vi "test SSL Client No Listener.vi"(8 "error in (no error)":errorcluster, 11 "TestCase in":refnum<class "test SSL Client.lvclass">) -> (0 "error out":errorcluster, 3 "TestCase out":refnum<class "test SSL Client.lvclass">)   [LabVIEW 2013, in "test SSL Client.lvclass"]
uses:
  test SSL Client.lvclass
  <vilib>/addons/_JKI Toolkits/VI Tester/TestCase.llb/TestCase.lvclass
  SSL_Lib/BIO/BIO.lvclass
  SSL_Lib/SSL-Context/SSL-Context.lvclass
  SSL_Lib/SSL/SSL.lvclass
  SSL_Lib/SSL/SSL_Mode.ctl
  suite SSL Client/suite SSL Client/SSL Context.vi
  suite SSL Client/suite SSL Client/suite SSL Client.lvclass
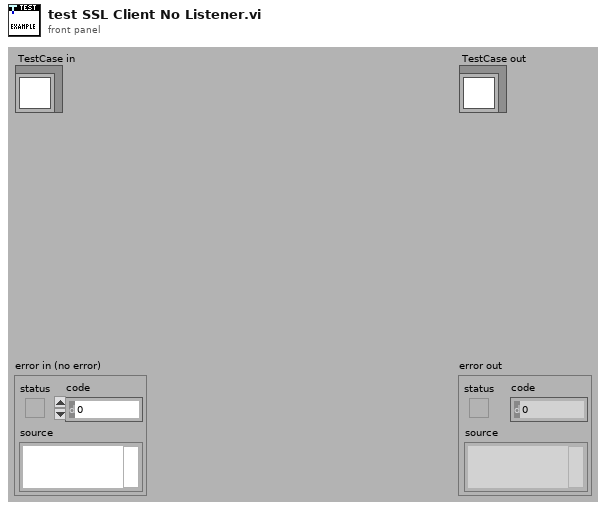
[diagram p1: front panel]
types:
  T1 = typedef "SSL_Lib.lvlib/SSL.lvclass/SSL_Mode.ctl" = i32
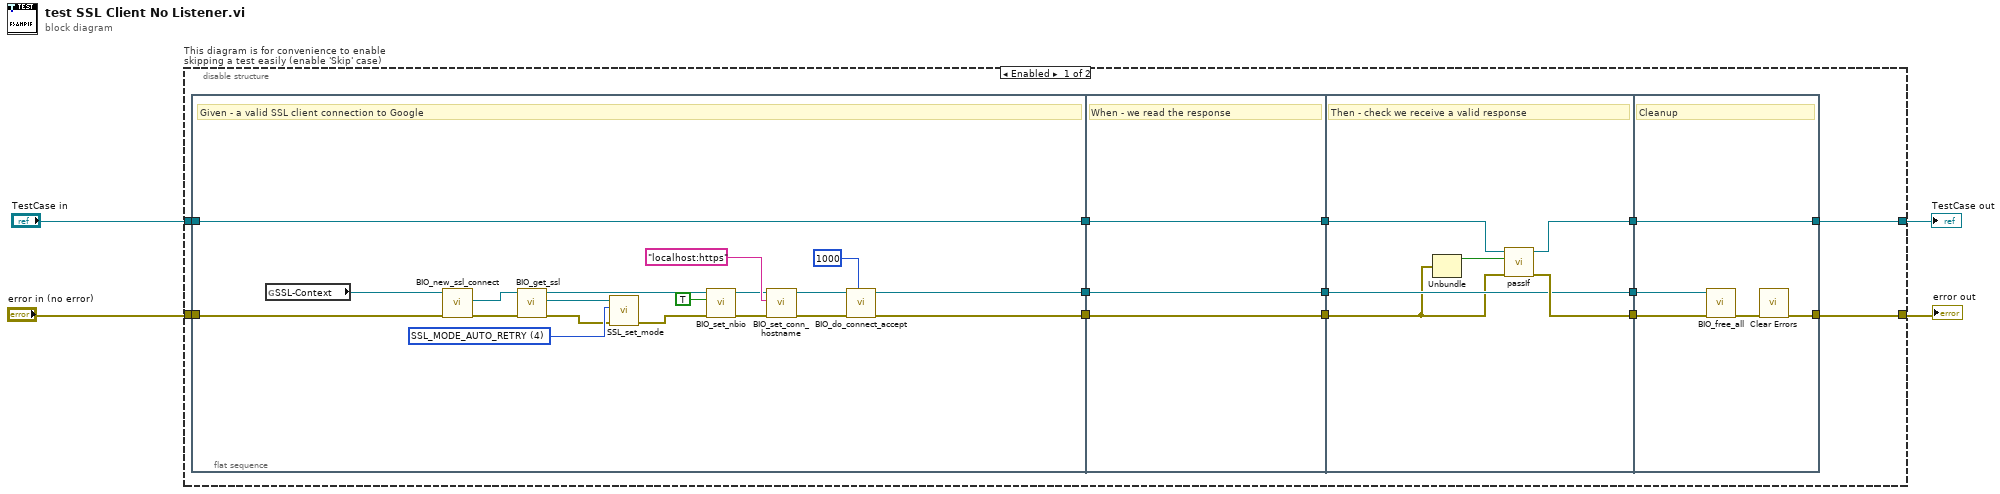
[diagram p0: block diagram]
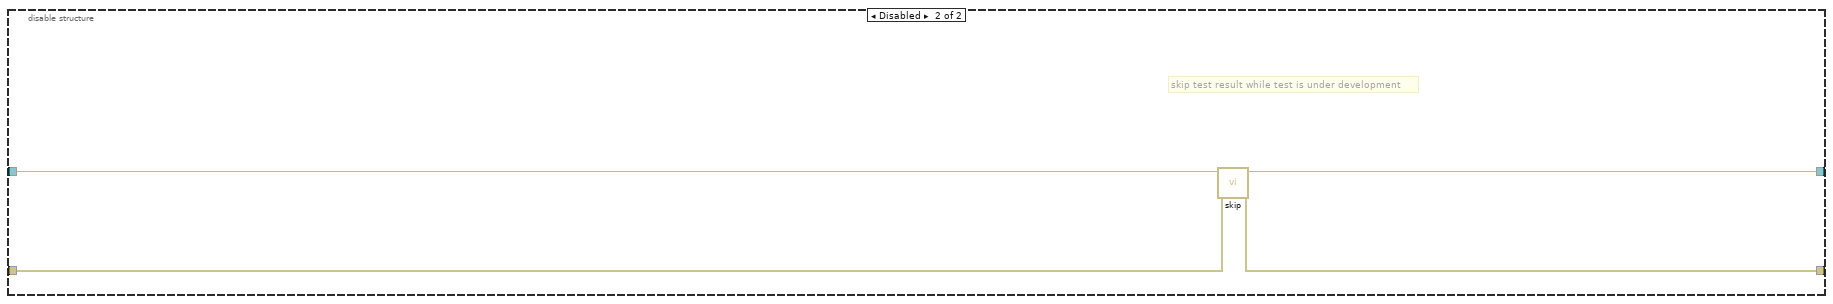
[diagram p2: hidden frame]
diagram:
  n1 = disable-structure "This diagram is for convenience to enable skipping a test easily (enable 'Skip' case)" shown="Enabled" {
    disable-tunnel: "TestCase in" -> [w12 w54]
    disable-tunnel: [w11 w52] -> w1
    disable-tunnel: [w10 w53] -> w3
    disable-tunnel: "error in (no error)" -> [w13 w51]
    frame Enabled {
      n2 = flat-sequence {
        tunnel: w13 -> [w26]
        tunnel: w12 -> [w33]
        tunnel: [w33] -> w17
        tunnel: [w19] -> w7
        tunnel: [w18] -> w6
        tunnel: [w39] -> w16
        tunnel: w17 -> [w39]
        tunnel: [w37] -> w9
        tunnel: w7 -> [w38]
        tunnel: w6 -> [w37]
        tunnel: [w38] -> w5
        tunnel: [w44] -> w15
        tunnel: [w43] -> w14
        tunnel: w16 -> [w45]
        tunnel: w9 -> [w42]
        tunnel: [w42] -> w8
        tunnel: w5 -> [w41]
        tunnel: [w46] -> w10
        tunnel: [w50] -> w11
        tunnel: w15 -> [w50]
        tunnel: w14 -> [w49]
        tunnel: w8 -> [w47]
        frame #0 {
          w28 = T1 4 items=["None"=0, "SSL_MODE_ENABLE_PARTIAL_WRITE"=1, "SSL_MODE_ACCEPT_MOVING_WRITE_BUFFER"=2, "SSL_MODE_AUTO_RETRY"=4, "SSL_MODE_RELEASE_BUFFERS"=16, "SSL_MODE_SEND_FALLBACK_SCSV"=128] ("Mode")
          # "Given - a valid SSL client connection to Google"
          n3 = global read "SSL Context.vi" "SSL-Context"() -> (w25:refnum<class "SSL-Context.lvclass">)
          n4 = call "BIO_new_ssl_connect.vi"("error in (no error)"=w26, "SSL-Context in"=w25) -> ("error out"=w30:errorcluster, "BIO out"=w31:refnum<class "BIO.lvclass">)  [unwired: 7 in, 1 out]
          n5 = call "BIO_get_ssl.vi"("error in (no error)"=w30, "BIO in"=w31) -> ("error out"=w27:errorcluster, "SSL out"=w29:refnum<class "SSL.lvclass">, "BIO out"=w20:refnum<class "BIO.lvclass">)  [unwired: 7 in]
          n6 = call "SSL_set_mode.vi"("error in (no error)"=w27, "Mode"=w28, "SSL in"=w29) -> ("error out"=w23:errorcluster)  [unwired: 7 in, 1 out]
          n7 = call "BIO_set_nbio.vi"("error in (no error)"=w23, "Non-Blocking?"=TRUE, "BIO in"=w20) -> ("error out"=w21:errorcluster, "BIO out"=w22:refnum<class "BIO.lvclass">)  [unwired: 7 in]
          n8 = call "BIO_set_conn_hostname.vi"("error in (no error)"=w21, "Hostname"="localhost:https", "BIO in"=w22) -> ("error out"=w35:errorcluster, "BIO out"=w32:refnum<class "BIO.lvclass">)  [unwired: 7 in]
          n9 = call "BIO_do_connect_accept.vi"("Timeout (10000ms)"=u32 1000, "error in (no error)"=w35, "BIO in"=w32) -> ("error out"=w19:errorcluster, "BIO out"=w18:refnum<class "BIO.lvclass">)  [unwired: 7 in]
        }
        frame #1 {
          # "When - we read the response"
        }
        frame #2 {
          # "Then - check we receive a valid response"
          n10 = Unbundle(w41) -> ("status"=w40:bool)  [unwired: 2 out]
          n11 = call-dynamic "passIf.vi"("error in (no error)"=w41, "pass"=w40, "TestCase in"=w45) -> ("error out"=w43:errorcluster, "TestCase out"=w44:refnum<class "test SSL Client.lvclass">)  [unwired: 7 in]
        }
        frame #3 {
          # "Cleanup"
          n12 = call "BIO_free_all.vi"("error in (no error)"=w49, "BIO in"=w47) -> ("error out"=w48:errorcluster)  [unwired: 9 in]
          n13 = call <vilib>:"Clear Errors.vi"("error in (no error)"=w48) -> ("error out"=w46:errorcluster)  [unwired: 5 in, 1 out]
        }
      }
    }
    frame Disabled {
      # "skip test result while test is under development"
      n14 = call <vilib>:"skip.vi"("error in (no error)"=w51, "TestCase in"=w54) -> ("error out"=w53:errorcluster, "TestCase out"=w52:refnum<class "test SSL Client.lvclass">)  [unwired: 8 in]
    }
  }
  "error out" <- w3
  "TestCase out" <- w1
